vi "HandShaking.vi"(6 "Elapsed Time":u32, 8 "error in (no error)":errorcluster, 10 "Event Sources":T1, 11 "OPC UA in":refnum<class "OPC UA.lvclass">) -> (0 "error out":errorcluster, 3 "OPC UA out":refnum<class "OPC UA.lvclass">)   [LabVIEW 2021, in "OPC UA.lvclass"]
uses:
  OPC UA.lvclass
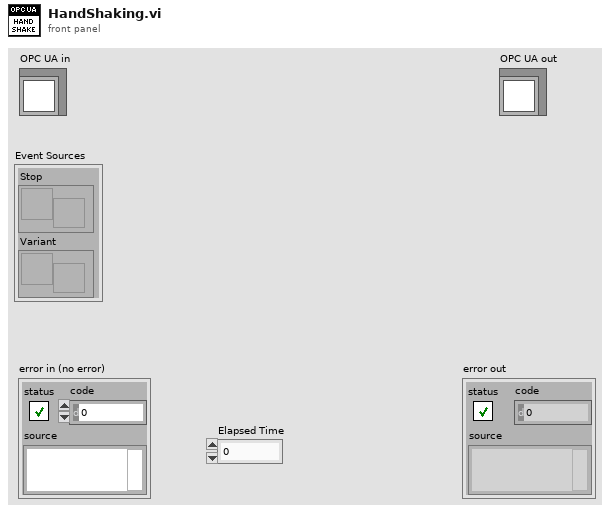
[diagram p1: front panel]
types:
  T1 = cluster{"Stop":refnum<user-event>, "Variant":refnum<user-event>}
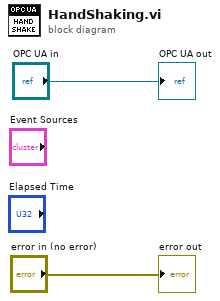
[diagram p0: block diagram]
diagram:
  "error out" <- "error in (no error)"
  "OPC UA out" <- "OPC UA in"
